vi "SetVisibillitySettings.vi"(0 "reference in":refnum<class "VINode.lvclass">, 1 "showAttribute":bool, 2 "showMethods":bool, 5 "error in (no error)":errorcluster) -> (14 "reference out":refnum<class "VINode.lvclass">, 19 "error out":errorcluster)   [LabVIEW 2016]
doc: "SetVisibillitySettings"
uses:
  <resource>/Framework/Providers/Open_GDS/UML/VINode_class/VINode.lvclass
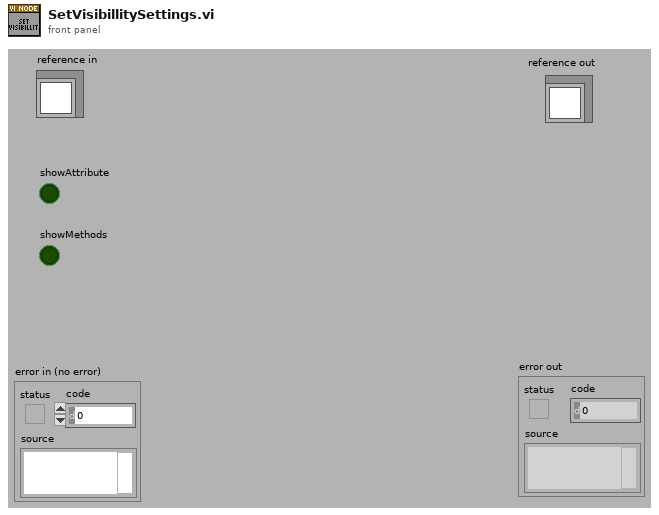
[diagram p1: front panel]
types:
  T1 = typedef "VINode.lvclass/ObjectAttributes.ctl" = cluster{"midHeight":dbl, "botHeight":dbl, "Name":refnum<class "MultiLineString.lvclass">, "DEFAULT_COMPARTMENT_HEIGHT":i32, "DEFAULT_WIDTH":i32, "DEFAULT_HEIGHT":i32, "VIPath":path, "Description":refnum<class "MultiLineString.lvclass">, "ShowDescription":bool}
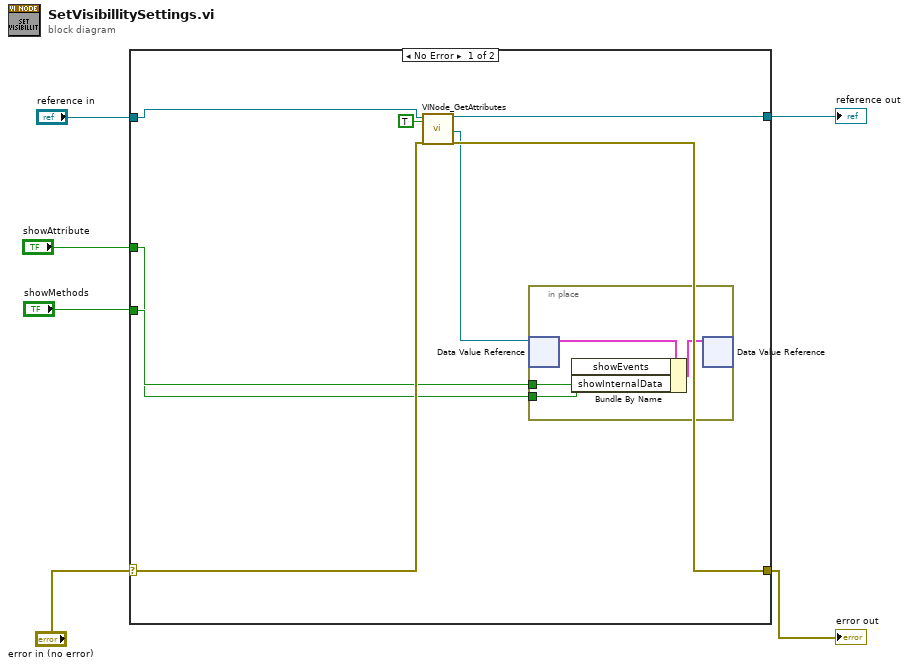
[diagram p0: block diagram]
diagram:
  n1 = case shown="No Error" "error in (no error)" {
    selector: "error in (no error)" -> [w14 w19]
    tunnel: "reference in" -> [w13 w20]
    tunnel: [w12 w19] -> w4
    tunnel: [w11 w20] -> w3
    tunnel: "showMethods" -> [w8 _]
    tunnel: "showAttribute" -> [w7 _]
    frame No Error {
      n2 = call <resource>:"VINode_GetAttributes.vi"("reference in"=w13, "OnlyGetDvrReference(False)"=TRUE, "error in (no error)"=w14) -> ("reference out"=w11:refnum<class "VINode.lvclass">, "DataRef"=w9:refnum<data-value>, "error out"=w12:errorcluster)  [unwired: 13 in, 1 out]
      n3 = in-place {
        in-place-border: w8 -> [w17]
        in-place-border: w7 -> [w16]
        n4 = in-place-dvr #1(w9) -> (w18:T1)  [unwired: 1 out]
        n5 = Bundle By Name(cluster=w18, "showEvents"=w17, "showInternalData"=w16) -> (w15:T1)
        n6 = in-place-dvr #1(w15) -> ()  [unwired: 2 out]
      }
    }
    frame Error {
    }
  }
  "reference out" <- w3
  "error out" <- w4
